vi "main.vi"() -> ()   [LabVIEW 2016]
panel:
  out "error out 2":errorcluster
  out "error out":errorcluster
  in  "vi path":path=path "D:/git/LabVIEW/ui-automation/labview-ui-testing/Prototype/ExeSubPanel/VI 2.vi"
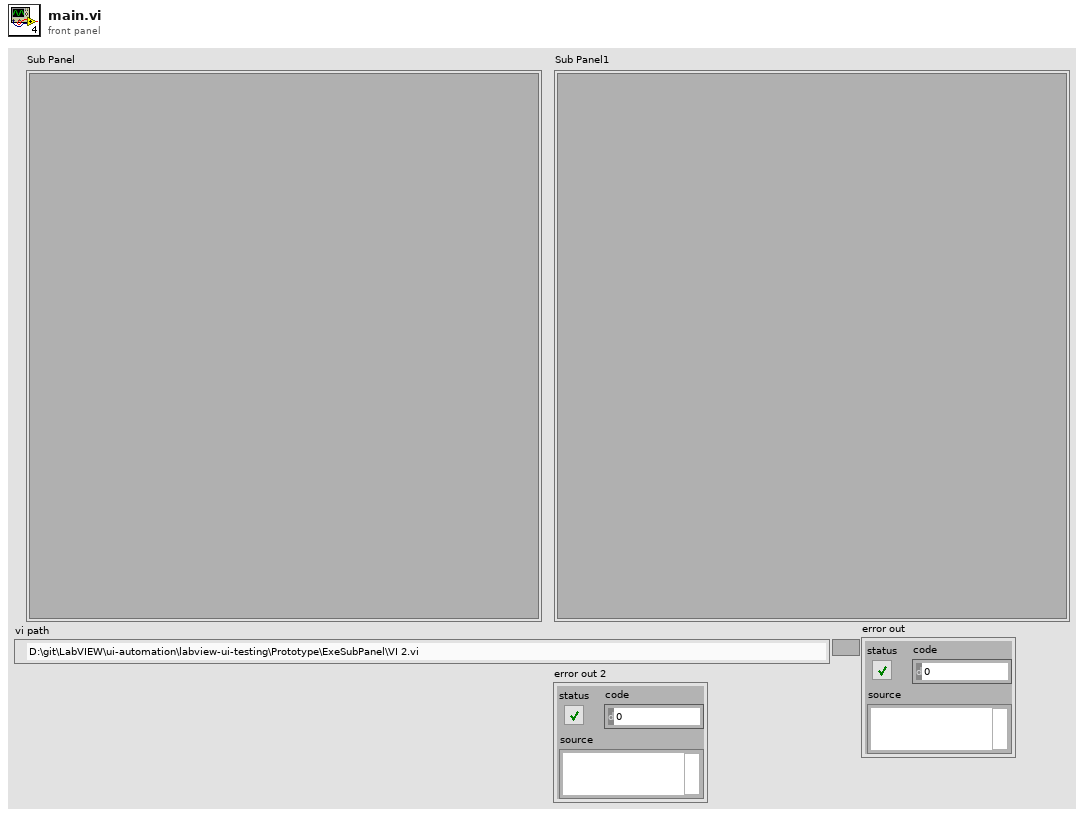
[diagram p1: front panel]
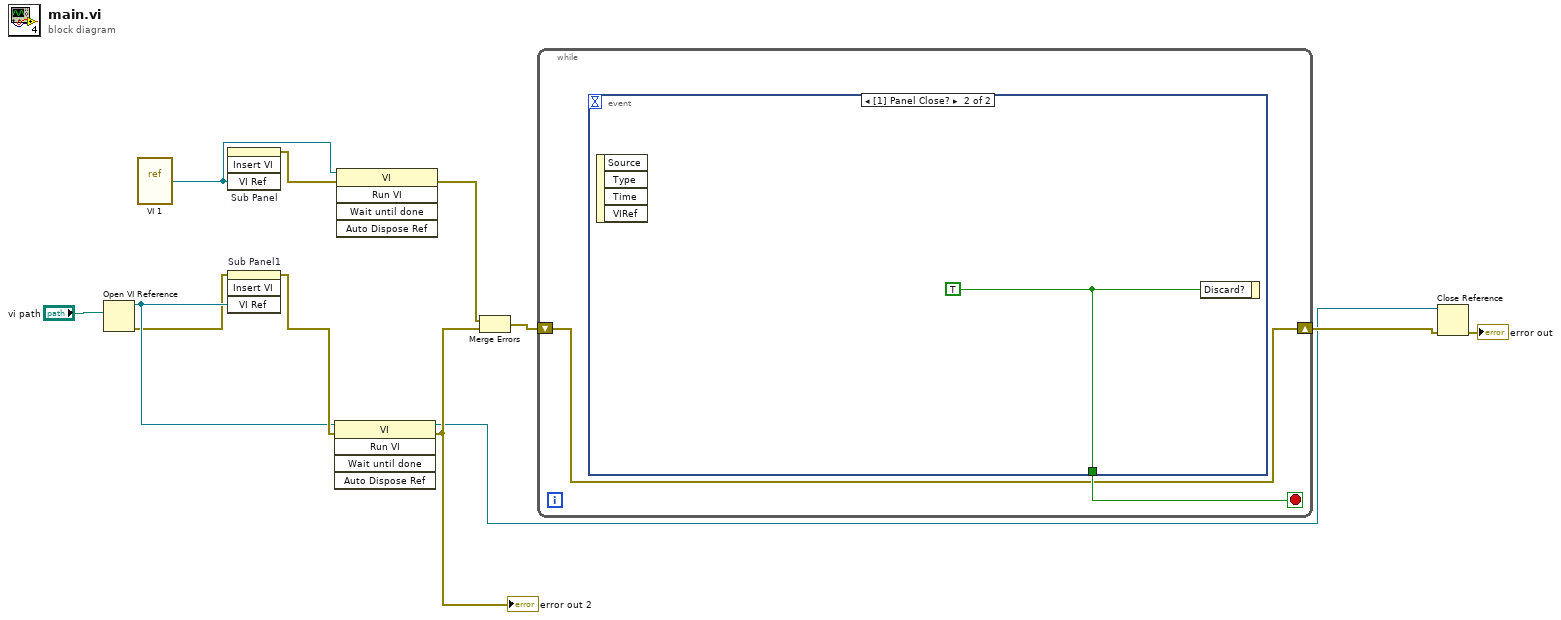
[diagram p0: block diagram]
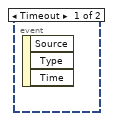
[diagram p2: hidden frame]
diagram:
  n1 = Open VI Reference(vi path="vi path") -> (vi reference=w5:refnum<vi>, error out=w4:errorcluster)  [unwired: 5 in]
  n2 = vi-ref "VI 1.vi"() -> (w12:refnum<vi>)
  n3 = invoke on="Sub Panel" class="SubPnl" method="Insert VI"("VI Ref"=w12) -> (error out=w11:errorcluster)  [unwired: 3 in, 3 out]
  n4 = invoke on="Sub Panel1" class="SubPnl" method="Insert VI"(error in=w4, "VI Ref"=w5) -> (error out=w8:errorcluster)  [unwired: 2 in, 3 out]
  n5 = invoke class="VI" method="Run VI"(reference=w5, error in=w8) -> (reference out=w6:refnum<vi>, error out=w7:errorcluster)  [unwired: 3 in, 3 out]
  "error out 2" <- w7
  n6 = invoke class="VI" method="Run VI"(reference=w12, error in=w11) -> (error out=w1:errorcluster)  [unwired: 3 in, 4 out]
  n7 = Merge Errors(w1, w7) -> (w2:errorcluster)
  n8 = while {
    shift-right: [w13] -> w9
    shift-left: w2 -> [w13]
    stop <- w14 stop-if-true
    n9 = event shown="[1] Panel Close?" {
      selector: _ -> [_ _]
      dyn-events: _ -> [_ _]
      timeout: _ -> [_ _]
      tunnel: [_ w15] -> w14
      event Timeout {
        n10 = event-data() -> ()  [unwired: 1 in, 3 out]
      }
      event Panel Close? {
        w15 = TRUE ("Discard?")
        n11 = event-data() -> ()  [unwired: 1 in, 4 out]
        n12 = event-data("Discard?"=w15) -> ()  [unwired: 1 in, 1 out]
      }
    }
  }
  n13 = Close Reference(reference=w6, error in (no error)=w9) -> (error out=→"error out":errorcluster)
